vi "TL Motor MoveAbsolute.vi"() -> ()   [LabVIEW 2021]
doc: "Shows how to move a motor to an absolute position."
panel:
  in  "MG17Motor":refnum<k7>(container)
  in  "Stop":bool
  in  "Set Abs Pos":bool
  in  "Abs Pos":dbl=1.0 min=-10.0 max=10.0 format="%.2f"
  in  "MoveAbsolute":bool
  in  "Home":bool
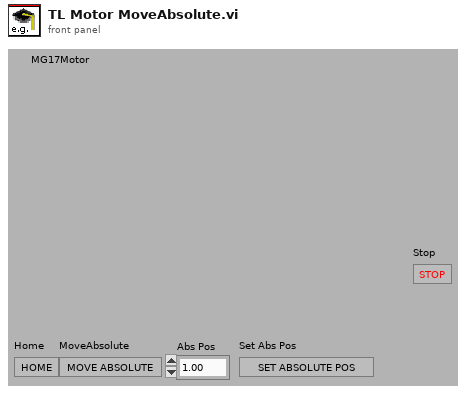
[diagram p1: front panel]
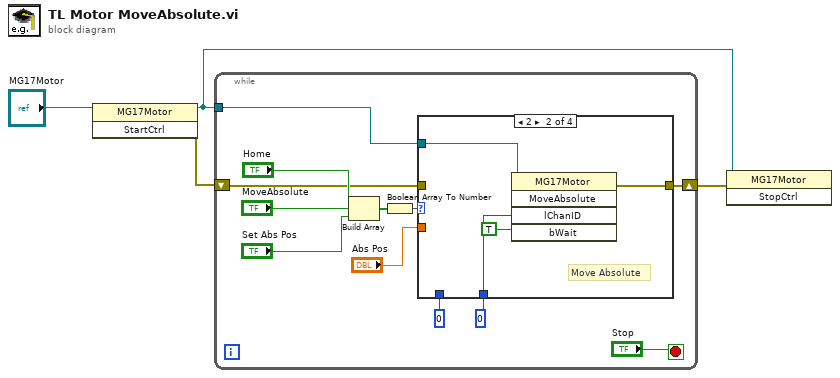
[diagram p0: block diagram]
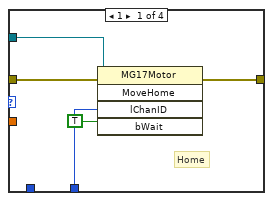
[diagram p2: hidden frame]
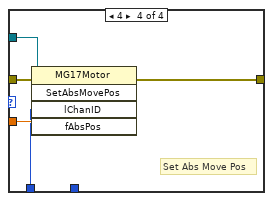
[diagram p4: hidden frame]
diagram:
  n1 = invoke class="MG17Motor" method="StartCtrl"(reference="MG17Motor") -> (reference out=w4:refnum<k7>, error out=w3:errorcluster)  [unwired: 2 in, 1 out]
  n2 = while {
    shift-left: w3 -> [w9]
    shift-right: [w10] -> w2
    tunnel: w4 -> [w14]
    stop <- "Stop" stop-if-true
    n3 = Build Array("Home", "MoveAbsolute", "Set Abs Pos") -> (w6:bool[])
    n4 = Boolean Array To Number(Boolean array=w6) -> (number=w7:u32)
    n5 = case shown="2" w7 {
      tunnel: w14 -> [w21 w25 _ w30]
      tunnel: 0 ("lChanID") -> [w20 w24 _ _]
      tunnel: "Abs Pos" -> [_ _ _ w29]
      tunnel: [w19 w23 w26 w27] -> w10
      tunnel: w9 -> [w18 _ w26 w31]
      tunnel: 0 ("lChanID") -> [_ _ _ w28]
      frame 1 {
        # "Home"
        n6 = invoke class="MG17Motor" method="MoveHome"(reference=w21, error in=w18, "lChanID"=w20, "bWait"=TRUE) -> (error out=w19:errorcluster)  [unwired: 1 in, 4 out]
      }
      frame 2 {
        # "Move Absolute"
        n7 = invoke class="MG17Motor" method="MoveAbsolute"(reference=w25, "lChanID"=w24, "bWait"=TRUE) -> (error out=w23:errorcluster)  [unwired: 2 in, 4 out]
      }
      frame Default {
      }
      frame 4 {
        # "Set Abs Move Pos"
        n8 = invoke class="MG17Motor" method="SetAbsMovePos"(reference=w30, error in=w31, "lChanID"=w28, "fAbsPos"=w29) -> (error out=w27:errorcluster)  [unwired: 1 in, 4 out]
      }
    }
  }
  n9 = invoke class="MG17Motor" method="StopCtrl"(reference=w4, error in=w2) -> ()  [unwired: 1 in, 3 out]
